vi "LinearBearingControl.vi"() -> ()   [LabVIEW 2012]
uses:
  stressTestTypeDef.ctl
  <vilib>/Utility/error.llb/DialogType.ctl
  allStatesTypeDef.ctl
  <vilib>/Utility/file.llb/Write To Spreadsheet File (DBL).vi
panel:
  out "sqrt(x)":dbl[](array[numeric])
  out "transposed array":dbl[][](array[numeric])
  in  "pulse/rev":u16(ring)=25600 items=["400"=400, "800"=800, "1600"=1600, "3200"=3200, "6400"=6400, "12800"=12800, "25600"=25600]
  out "concatenated string":string
  out "rigid body LED":bool
  out "strain rate":dbl
  in  "chain L0":i32=230
  out "mm/s (timed)":dbl
  in  "Direction":bool
  in  "Only Move Lin":bool
  out "writing data":bool
  out "stop sys":bool
  out "udp error out":errorcluster
  out "Voltages":dbl[][](array[numeric])
  in  "Start System":bool
  in  "Auto Bias":bool=TRUE
  in  "Unbias":bool
  in  "Bias":bool
  in  "Collect Data":bool=TRUE
  out "Measurement":dbl[][](graph) caption="F/T Data"
  out "Bias Vector":dbl[](array[numeric])
  in  "Timing parameters":T1={"Sample Rate"=1000.0, "Samples to Read"=100}
  in  "Transform":T2
  in  "Channel Parameters":T3={"First Channel"=1, "Number of Channels"=6, "DAQ Card"="Dev2", "Maximum Value"=10.0, "Minimum Value"=-10.0}
  in  "Sensor Parameters":T4={"Calibration File"=path "D:/ArduinoSmarticle/entangledSmarticle/FT21164.cal", "Force Units"="N", "Torque Units"="N-mm"}
  out "filenameOut":string
  in  "Optitrack Parameters":T5={"Optitrack IP"="130.207.141.229", "Optitrack Port"=1520, "timeout (sec)"=80}
  out "Data Output File":path
  in  "Output Folder":path=path "C:/Users/Administrator/Dropbox/expData/chainData"
  in  "Program Parameters":T7={"v"=2200, "Iters"=2, "Speed"=5, "Delay"=0.5, "H"=11.5, "SD"=10, "Name"="Stretch", "Type"=enum."FRACT ON"} {"Speed" min=0 max=49 step=5}
  out "strain %":dbl
  out "FT error out":errorcluster
  # "for 6 smarts\nSDmax ~ 170mm"
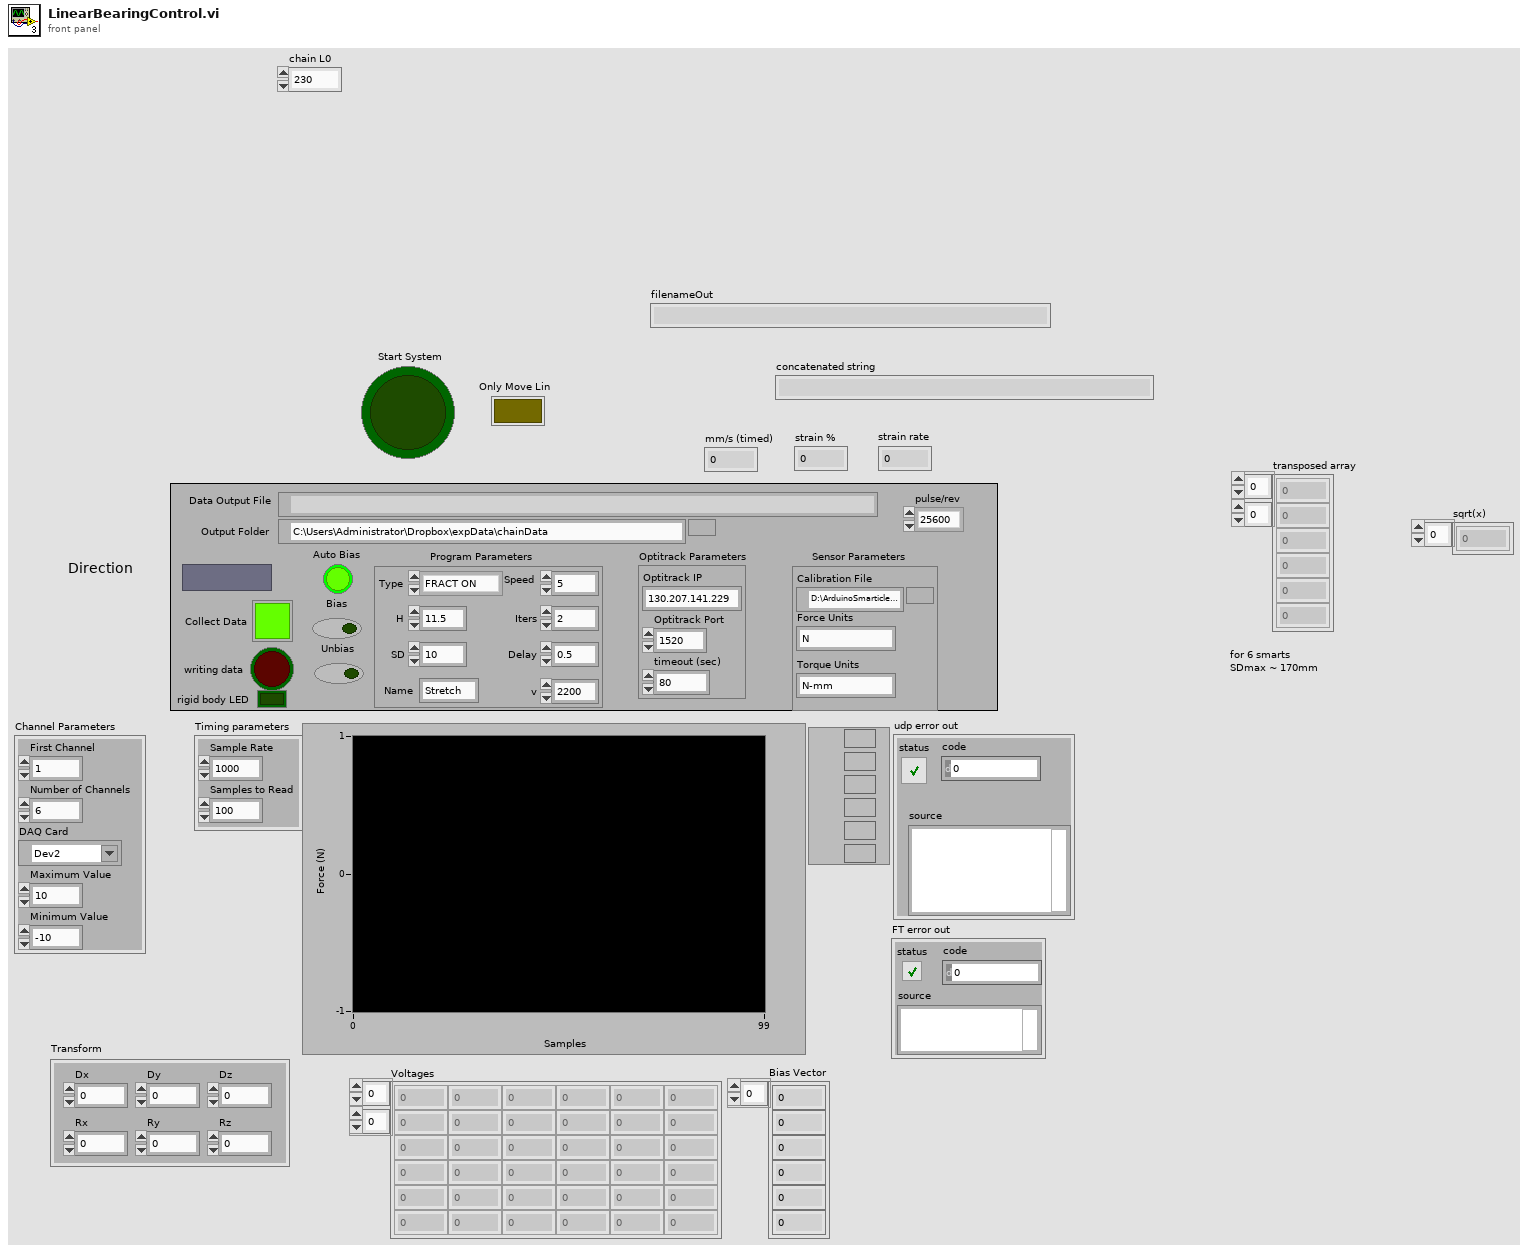
[diagram p1: front panel]
types:
  T1 = cluster{"Sample Rate":dbl, "Samples to Read":i32}
  T2 = cluster{"Dx":dbl, "Dy":dbl, "Dz":dbl, "Rx":dbl, "Ry":dbl, "Rz":dbl}
  T3 = cluster{"First Channel":i16, "Number of Channels":i16, "DAQ Card":tag, "Maximum Value":dbl, "Minimum Value":dbl}
  T4 = cluster{"Calibration File":path, "Force Units":string, "Torque Units":string}
  T5 = cluster{"Optitrack IP":string, "Optitrack Port":u16, "timeout (sec)":i32}
  T6 = typedef "stressTestTypeDef.ctl" = enum16{"OFF", "ON", "EXTEND", "SPRING", "FRACT ON", "SAC", "FRACT SAC"}
  T7 = cluster{"v":i32, "Iters":i32, "Speed":i32, "Delay":dbl, "H":dbl, "SD":i32, "Name":string, "Type":T6}
  T8 = cluster{"distance mm":i32, "Direction":bool, "device name":tag, "speed (mm/s)":i32, "pulse/rev":u16}
  T9 = typedef "DialogType.ctl" = u16
  T10 = cluster{"SD":i32, "Delay":dbl, "Speed":i32, "Iters":i32, "Type":T6, "timeout":i32}
  T11 = typedef "allStatesTypeDef.ctl" = enum16{"open udp", "start record", "recording", "move linear actuator", "end record", "close udp", "end"}
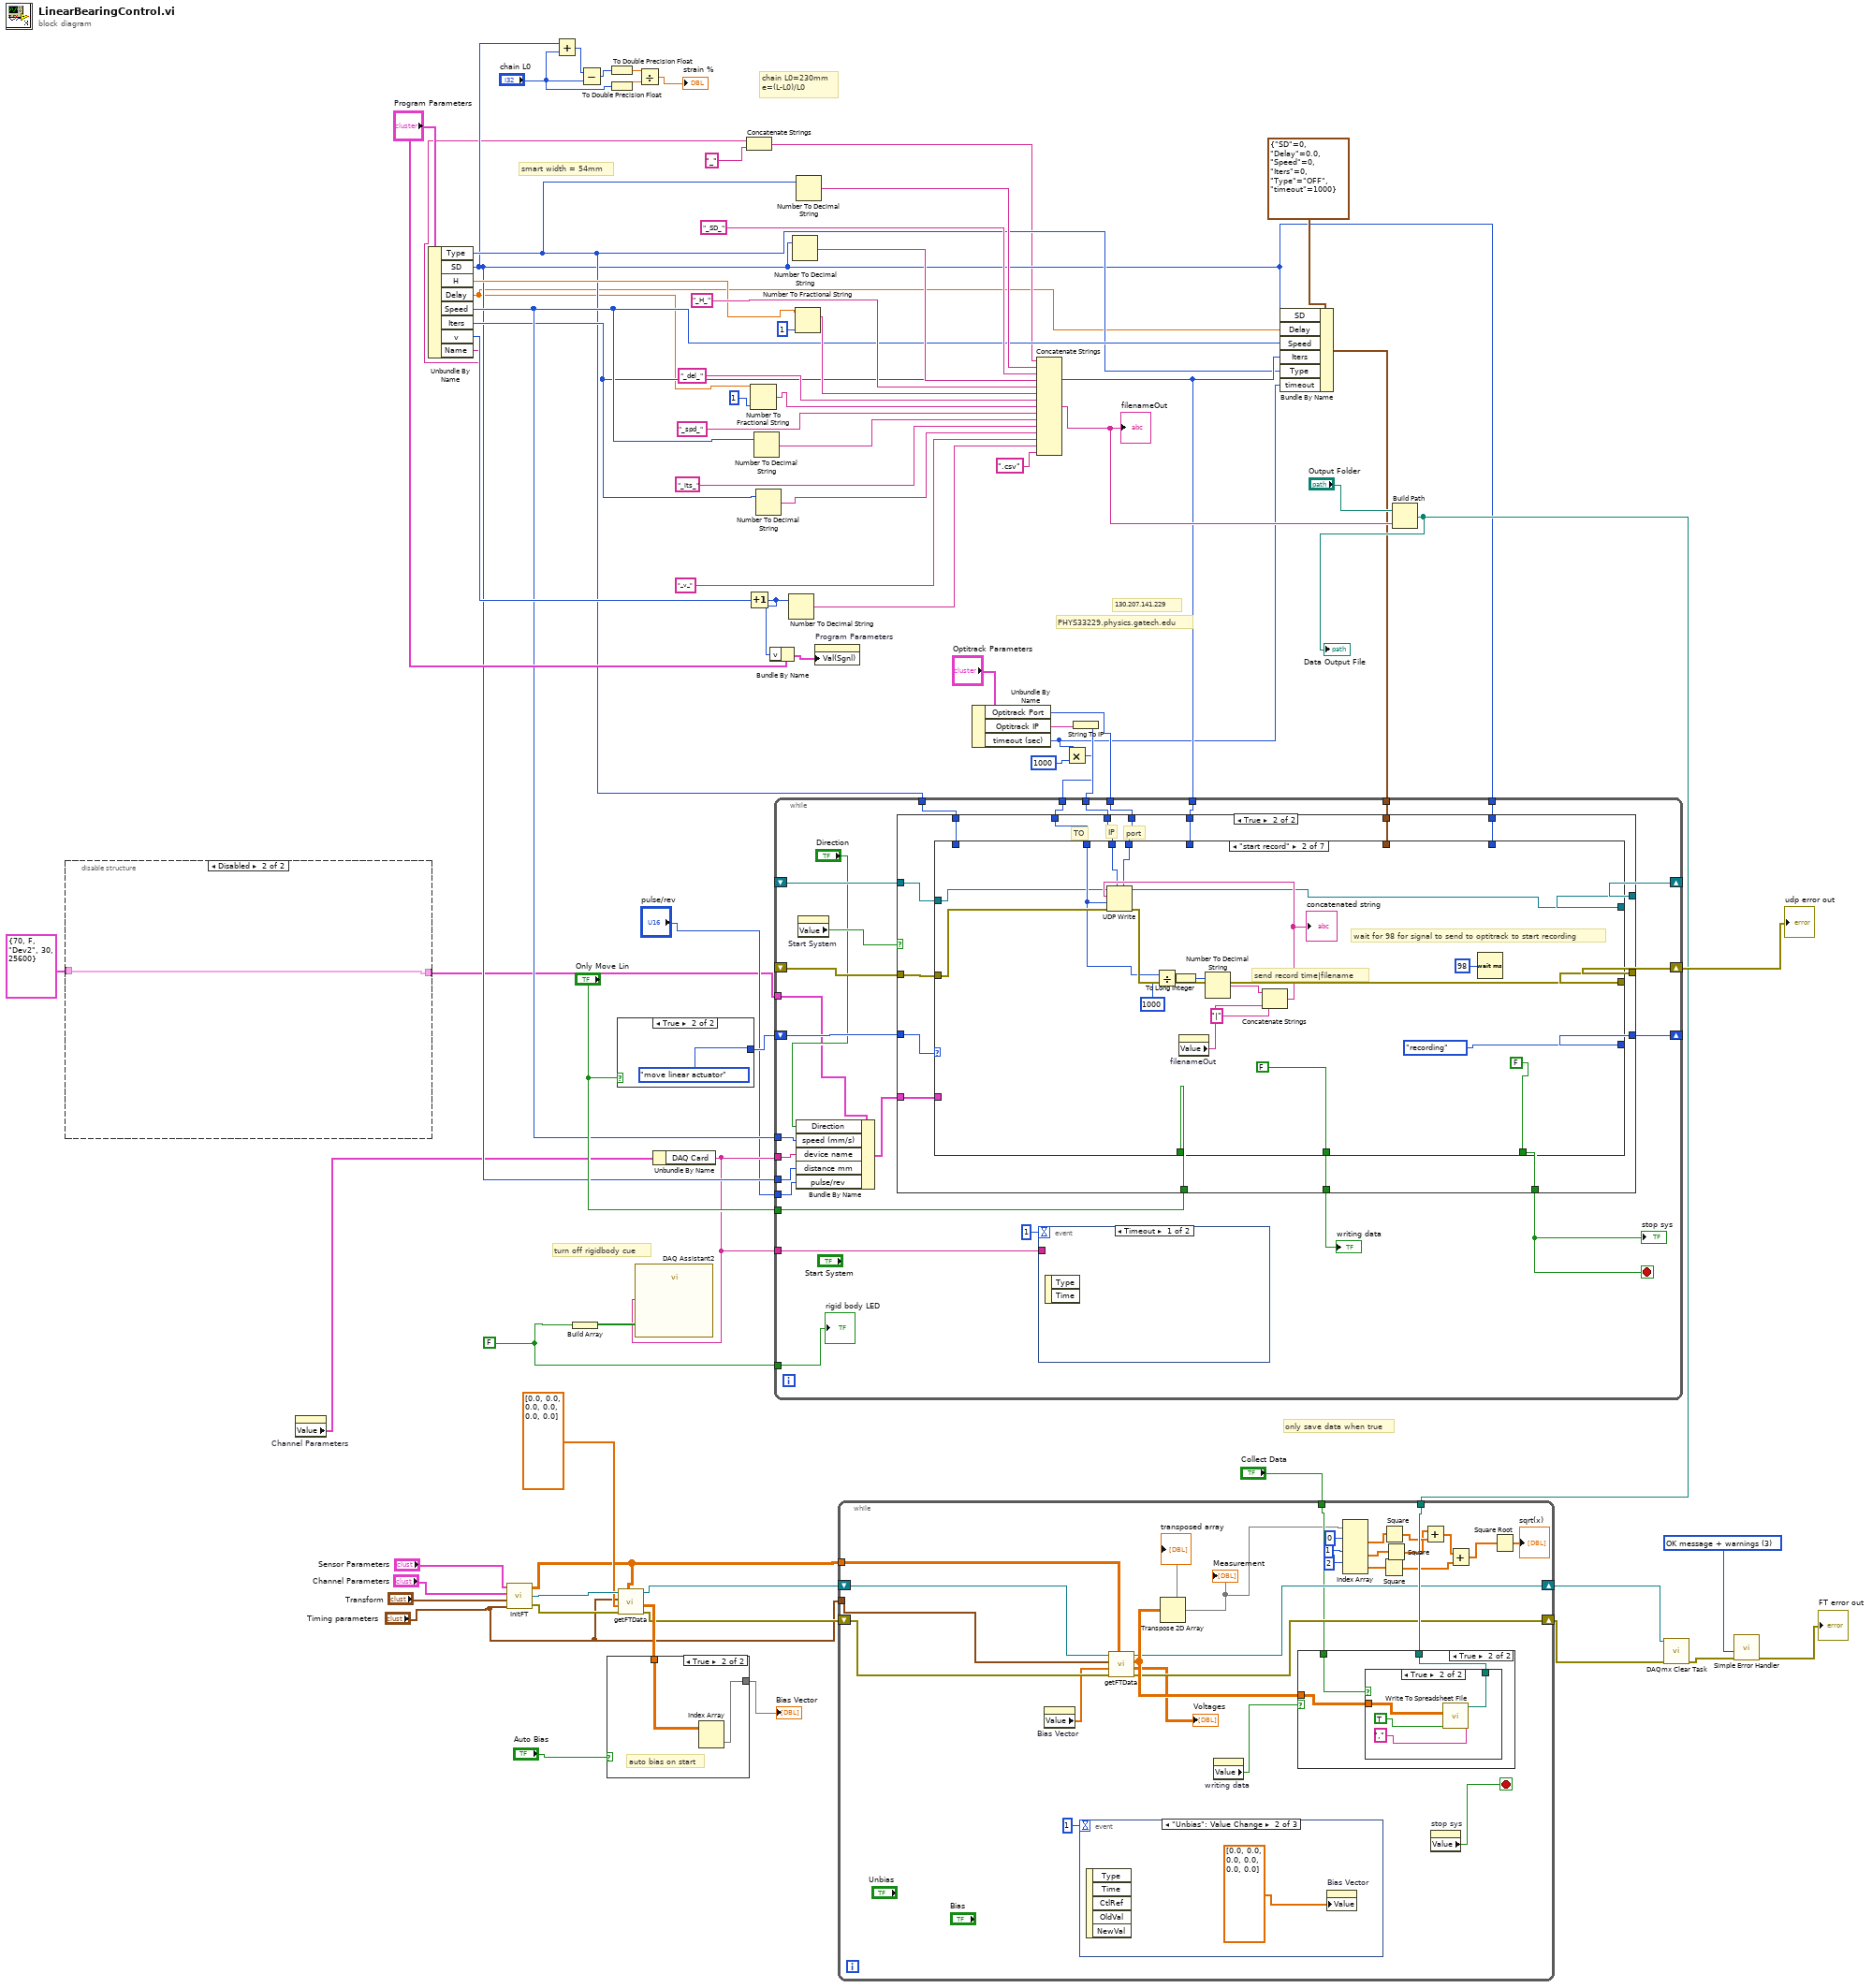
[diagram p0: block diagram]
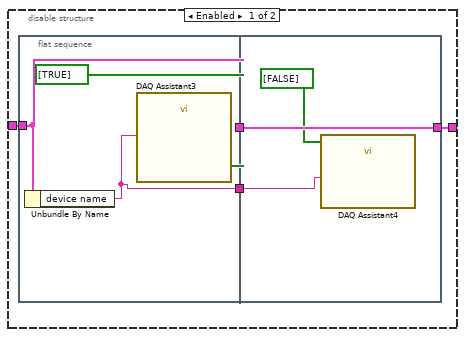
[diagram p2: hidden frame]
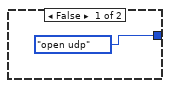
[diagram p3: hidden frame]
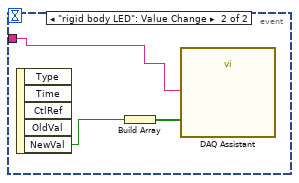
[diagram p4: hidden frame]
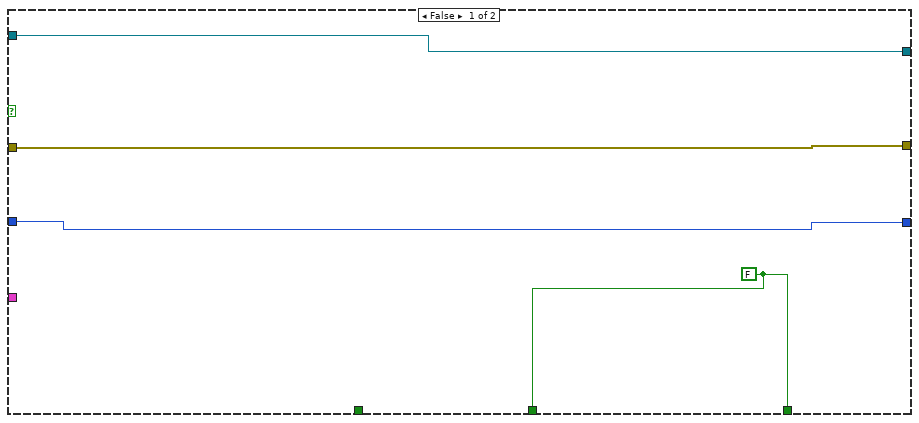
[diagram p5: hidden frame]
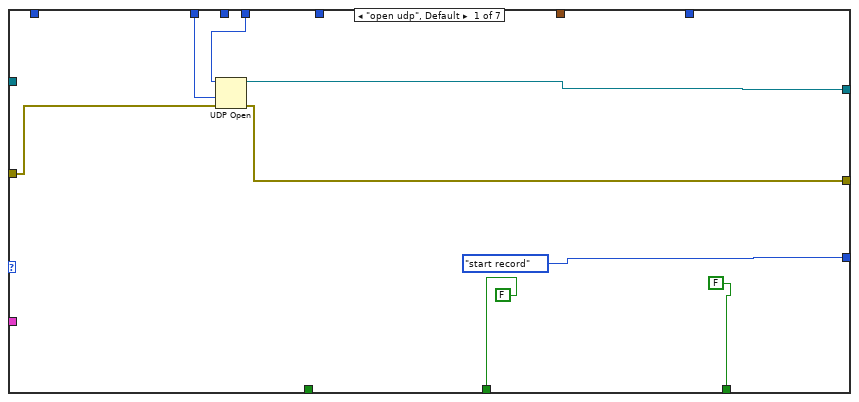
[diagram p6: hidden frame]
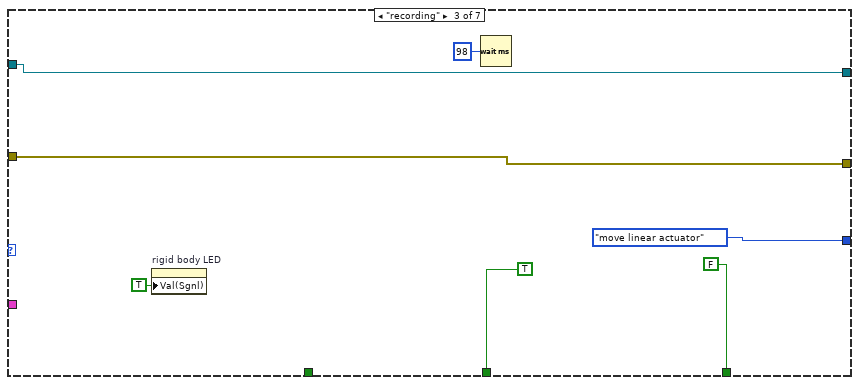
[diagram p7: hidden frame]
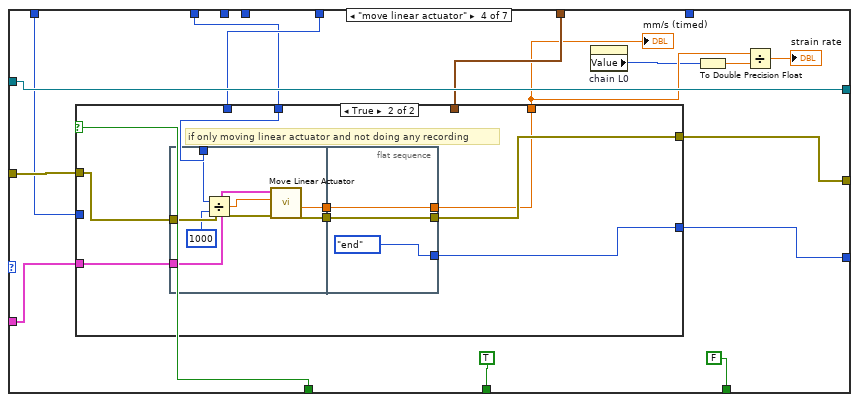
[diagram p8: hidden frame]
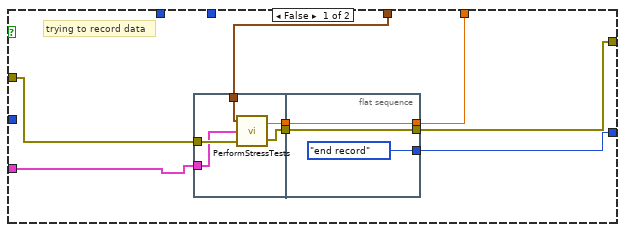
[diagram p9: hidden frame]
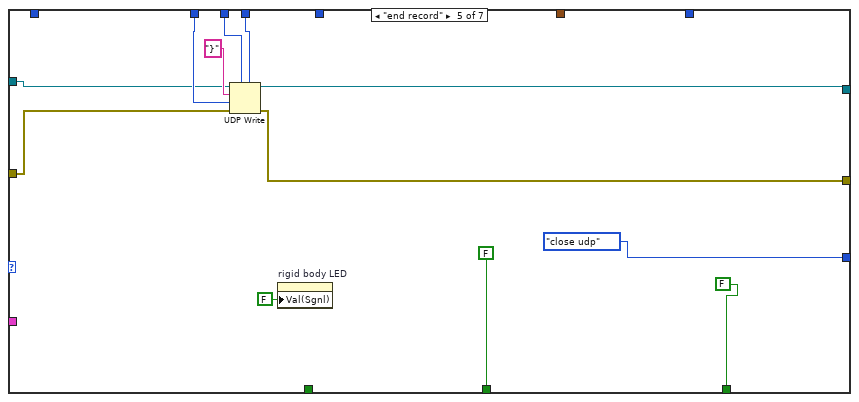
[diagram p10: hidden frame]
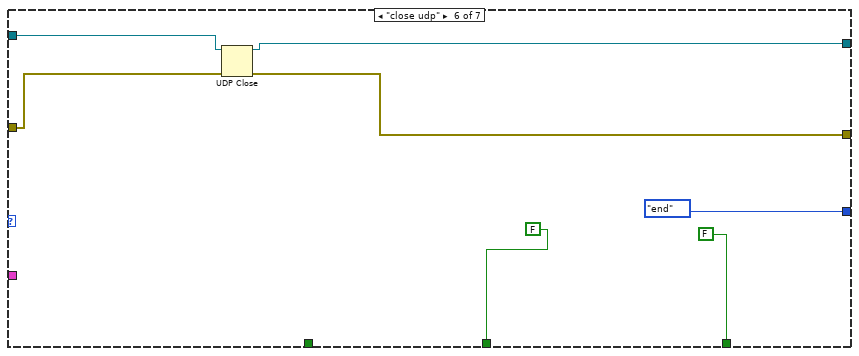
[diagram p11: hidden frame]
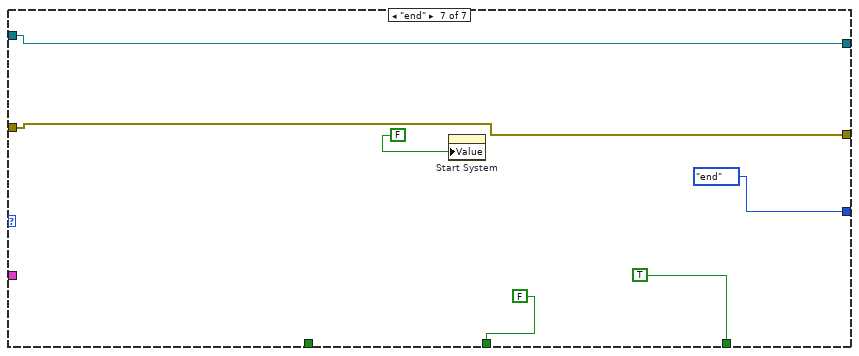
[diagram p12: hidden frame]
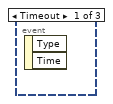
[diagram p13: hidden frame]
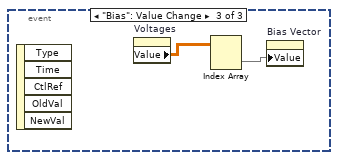
[diagram p14: hidden frame]
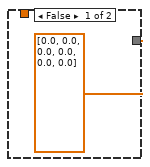
[diagram p17: hidden frame]
diagram:
  w13 = FALSE
  w46 = T9 3 items=["no dialog", "OK message", "continue or stop message", "OK message + warnings", "continue/stop + warnings"] ("type of dialog (OK msg:1)")
  # "turn off rigidbody cue"
  # "chain L0=230mm\ne=(L-L0)/L0"
  # "only save data when true"
  # "smart width = 54mm"
  # "PHYS33229.physics.gatech.edu"
  # "130.207.141.229"
  n1 = disable-structure shown="Disabled" {
    disable-tunnel: [w78 w87] -> w2
    disable-tunnel: T8 {"distance mm"=70, "Direction"=FALSE, "device name"="Dev2", "speed (mm/s)"=30, "pulse/rev"=25600} ("linear actuator info") -> [w77 w87]
    frame Enabled {
      n2 = flat-sequence {
        tunnel: w77 -> [w83]
        tunnel: [w83] -> w80
        tunnel: [w81] -> w79
        tunnel: [w86] -> w78
        tunnel: w80 -> [w86]
        tunnel: w79 -> [w85]
        frame #0 {
          n3 = Unbundle By Name(w83) -> ("device name"=w81:tag)
          n4 = call "DAQ Assistant3"("data"=bool[] [TRUE], "device name"=w81) -> ()  [unwired: 16 in, 2 out]
        }
        frame #1 {
          n5 = call "DAQ Assistant4"("data"=bool[] [FALSE], "device name"=w85) -> ()  [unwired: 16 in, 2 out]
        }
      }
    }
    frame Disabled {
    }
  }
  n6 = property on="Channel Parameters" class="Clust (strict)"() -> ("Value"=w12:T3)  [unwired: 2 in, 2 out]
  n7 = Unbundle By Name("Program Parameters") -> ("Type"=w23:T6, "SD"=w15:i32, "H"=w58:dbl, "Delay"=w5:dbl, "Speed"=w25:i32, "Iters"=w24:i32, "v"=w59:i32, "Name"=w8:string)
  n8 = call "InitFT.vi"("Timing parameters"="Timing parameters", "Transform"="Transform", "Channel Parameters"="Channel Parameters", "Sensor Parameters"="Sensor Parameters") -> ("error out"=w42:errorcluster, "task out"=w43:refnum<k21>, "Calibration Matrix"=w37:dbl[][])
  n9 = Add(x=w15, y="chain L0") -> (x+y=w21:i32)
  n10 = Build Array(w13) -> (w14:bool[])
  n11 = Subtract(x=w21, y="chain L0") -> (x-y=w20:i32)
  n12 = To Double Precision Float(number=w20) -> (double precision float=w18:dbl)
  n13 = To Double Precision Float(number="chain L0") -> (double precision float=w17:dbl)
  n14 = case shown="True" "Only Move Lin" {
    tunnel: [allStatesTypeDef."open udp" allStatesTypeDef."move linear actuator"] -> w76
    frame False {
    }
    frame True {
    }
  }
  n15 = call "getFTData.vi"("Transformed Calibration Matrix"=w37, "error in"=w42, "Bias Vector"=dbl[] [0.0, 0.0, 0.0, 0.0, 0.0, 0.0], "Timing parameters"="Timing parameters", "task in"=w43) -> ("error out"=w35:errorcluster, "Voltages"=w40:dbl[][], "task out 2"=w36:refnum<k21>)  [unwired: 1 out]
  n16 = case shown="True" "Auto Bias" {
    tunnel: w40 -> [_ w92]
    tunnel: [dbl[] [0.0, 0.0, 0.0, 0.0, 0.0, 0.0] w91] -> w33
    frame False {
    }
    frame True {
      # "auto bias on start"
      n17 = Index Array(array=w92) -> (element=w91:dbl[])  [unwired: 2 in]
    }
  }
  "Bias Vector" <- w33
  n18 = Divide(x=w18, y=w17) -> (x/y=→"strain %":dbl)
  n19 = Unbundle By Name(w12) -> ("DAQ Card"=w11:tag)
  n20 = call "DAQ Assistant2"("data"=w14, "device name"=w11) -> ()  [unwired: 16 in, 2 out]
  n21 = Concatenate Strings(w8, "_") -> (w9:string)
  n22 = Increment(x=w59) -> (x+1=w60:i32)
  n23 = Number To Fractional String(number=w5, precision (6)=i16 1) -> (F-format string=w3:string)  [unwired: 2 in]
  n24 = Number To Decimal String(number=w25) -> (decimal integer string=w64:string)  [unwired: 1 in]
  n25 = Number To Decimal String(number=w24) -> (decimal integer string=w62:string)  [unwired: 1 in]
  n26 = Bundle By Name(cluster="Program Parameters", "v"=w60) -> (w56:T7)
  n27 = Number To Decimal String(number=w60) -> (decimal integer string=w66:string)  [unwired: 1 in]
  n28 = Number To Decimal String(number=w15) -> (decimal integer string=w72:string)  [unwired: 1 in]
  n29 = Number To Fractional String(number=w58, precision (6)=i16 1) -> (F-format string=w69:string)  [unwired: 2 in]
  n30 = Number To Decimal String(number=w23) -> (decimal integer string=w74:string)  [unwired: 1 in]
  n31 = property on="Program Parameters" class="Clust (strict)"("Val(Sgnl)"=w56) -> ()  [unwired: 2 in, 2 out]
  n32 = Unbundle By Name("Optitrack Parameters") -> ("Optitrack Port"=w54:u16, "Optitrack IP"=w53:string, "timeout (sec)"=w7:i32)
  n33 = Concatenate Strings(w9, w74, "_SD_", w72, "_H_", w69, "_del_", w3, "_spd_", w64, "_its_", w62, "_v_", w66, ".csv") -> (w27:string)
  "filenameOut" <- w27
  n34 = Multiply(x=w7, y=1000) -> (x*y=w50:i32)
  n35 = String To IP(1:w53) -> (0:w52:u32)
  n36 = Bundle By Name(cluster=T10 {"SD"=0, "Delay"=0.0, "Speed"=0, "Iters"=0, "Type"=enum."OFF", "timeout"=1000}, "SD"=w15, "Delay"=w5, "Speed"=w25, "Iters"=w24, "Type"=w23, "timeout"=w7) -> (w22:T10)
  n37 = while {
    shift-right: [w119] -> w30
    shift-left: _ -> [w118]
    shift-right: [w116] -> _
    shift-left: w76 -> [w117]
    tunnel: w54 -> [w114]
    tunnel: w52 -> [w115]
    tunnel: w50 -> [w95]
    shift-right: [w113] -> _
    shift-left: _ -> [w112]
    tunnel: "Only Move Lin" -> [w109]
    tunnel: w25 -> [w106]
    tunnel: w15 -> [w97]
    tunnel: w23 -> [w105]
    tunnel: w24 -> [w104]
    tunnel: w22 -> [w103]
    tunnel: w15 -> [w101]
    tunnel: w13 -> [w100]
    tunnel: w11 -> [w98]
    tunnel: w11 -> [w96]
    tunnel: "pulse/rev" -> [w94]
    tunnel: w2 -> [w93]
    stop <- w111 stop-if-true
    n38 = Bundle By Name(cluster=w93, "Direction"="Direction", "speed (mm/s)"=w106, "device name"=w98, "distance mm"=w97, "pulse/rev"=w94) -> (w108:T8)
    n39 = property on="Start System" class="Bool (strict)"() -> ("Value"=w110:bool)  [unwired: 2 in, 2 out]
    n40 = case shown="True" w110 {
      tunnel: [w123 w143] -> w119
      tunnel: w118 -> [w123 w142]
      tunnel: w117 -> [w126 w141]
      tunnel: [w126 w140] -> w116
      tunnel: w115 -> [_ w139]
      tunnel: w114 -> [_ w132]
      tunnel: w95 -> [_ w138]
      tunnel: [w124 w137] -> w113
      tunnel: w112 -> [w124 w136]
      tunnel: [w125 w135] -> w102
      tunnel: [w125 w134] -> w111
      tunnel: w109 -> [_ w133]
      tunnel: w108 -> [_ w131]
      tunnel: w105 -> [_ w130]
      tunnel: w104 -> [_ w129]
      tunnel: w103 -> [_ w128]
      tunnel: w101 -> [_ w127]
      frame False {
        w125 = FALSE
      }
      frame True {
        # "IP"
        # "TO"
        # "port"
        n41 = case shown="\"start record\"" w141 {
          tunnel: w138 -> [w148 w161 _ w177 w234 _ _]
          tunnel: w142 -> [w149 w167 w172 w188 w238 w244 w246]
          tunnel: [w150 w168 w172 w187 w237 w245 w246] -> w143
          tunnel: [allStatesTypeDef."start record" allStatesTypeDef."recording" allStatesTypeDef."move linear actuator" w190 allStatesTypeDef."close udp" allStatesTypeDef."end" allStatesTypeDef."end"] -> w140
          tunnel: [FALSE FALSE FALSE FALSE FALSE FALSE TRUE] -> w134
          tunnel: w139 -> [_ w154 _ _ w228 _ _]
          tunnel: [w147 w157 w173 w189 w232 w243 w251] -> w137
          tunnel: w136 -> [_ w158 w173 w189 w231 w239 w251]
          tunnel: [FALSE FALSE TRUE TRUE FALSE FALSE FALSE] -> w135
          tunnel: w133 -> [_ _ _ w186 _ _ _]
          tunnel: w132 -> [w144 w153 _ _ w229 _ _]
          tunnel: w131 -> [_ _ _ w185 _ _ _]
          tunnel: w130 -> [_ _ _ w183 _ _ _]
          tunnel: w129 -> [_ _ _ w184 _ _ _]
          tunnel: w128 -> [_ _ _ w182 _ _ _]
          tunnel: w127 -> [_ _ _ _ _ _ _]
          frame "open udp", Default {
            n42 = UDP Open(8:w149, 9:w148, 11:w144) -> (port=w147:refnum<k16>, 0:w150:errorcluster)  [unwired: 2 in, 1 out]
          }
          frame "start record" {
            # "wait for 98 for signal to send to optitrack to start recording"
            # "send record time|filename"
            n43 = Divide(x=w161, y=1000) -> (x/y=w160:dbl)
            n44 = To Long Integer(number=w160) -> (32bit integer=w159:i32)
            n45 = property on="filenameOut" class="Str"() -> ("Value"=w165:string)  [unwired: 2 in, 2 out]
            n46 = Number To Decimal String(number=w159) -> (decimal integer string=w163:string)  [unwired: 1 in]
            n47 = Concatenate Strings(w163, "|" ("string"), w165) -> (w164:string)
            "concatenated string" <- w164
            n48 = UDP Write(address=w154, port or service name=w153, connection ID=w158, data in=w164, 8:w167, 9:w161) -> (error out=w168:errorcluster, 3:w157:refnum<k16>)
            n49 = Wait (ms)(milliseconds to wait=u32 98) -> ()  [unwired: 1 out]
          }
          frame "recording" {
            n50 = property on="rigid body LED" class="Bool (strict)"("Val(Sgnl)"=TRUE ("Value (Signaling)")) -> ()  [unwired: 2 in, 2 out]
            n51 = Wait (ms)(milliseconds to wait=u32 98) -> ()  [unwired: 1 out]
          }
          frame "move linear actuator" {
            n52 = case shown="True" w186 {
              tunnel: [w193 w210] -> w190
              tunnel: w188 -> [w197 w214]
              tunnel: [w196 w215] -> w187
              tunnel: w185 -> [w198 w216]
              tunnel: [w199 w213] -> w181
              tunnel: w184 -> [_ _]
              tunnel: w183 -> [_ _]
              tunnel: w182 -> [w200 _]
              tunnel: w177 -> [_ w209]
              frame False {
                # "trying to record data"
                n53 = flat-sequence {
                  tunnel: w200 -> [w205]
                  tunnel: w198 -> [w201]
                  tunnel: w197 -> [w203]
                  tunnel: [w204] -> w195
                  tunnel: [w202] -> w194
                  tunnel: w195 -> [w208]
                  tunnel: w194 -> [w207]
                  tunnel: [w208] -> w199
                  tunnel: [w207] -> w196
                  tunnel: [allStatesTypeDef."end record"] -> w193
                  frame #0 {
                    n54 = call "PerformStressTests.vi"("error in"=w203, "linear actuator info"=w201, "Test Info"=w205) -> ("error out"=w202:errorcluster, "mm/s (timed)"=w204:dbl)
                  }
                  frame #1 {
                  }
                }
              }
              frame True {
                # "if only moving linear actuator and not doing any recording"
                n55 = flat-sequence {
                  tunnel: w216 -> [w223]
                  tunnel: w214 -> [w221]
                  tunnel: [w222] -> w212
                  tunnel: [w220] -> w211
                  tunnel: w209 -> [w218]
                  tunnel: w212 -> [w226]
                  tunnel: w211 -> [w225]
                  tunnel: [w226] -> w215
                  tunnel: [w225] -> w213
                  tunnel: [allStatesTypeDef."end"] -> w210
                  frame #0 {
                    n56 = Divide(x=w218, y=1000) -> (x/y=w217:dbl)
                    n57 = call "Move Linear Actuator.vi"("error in"=w221, "timeout"=w217, "linear actuator info"=w223) -> ("error out"=w222:errorcluster, "mm/s (timed)"=w220:dbl)  [unwired: 1 in, 1 out]
                  }
                  frame #1 {
                  }
                }
              }
            }
            "mm/s (timed)" <- w181
            n58 = property on="chain L0" class="DigNum (strict)"() -> ("Value"=w180:i32)  [unwired: 2 in, 2 out]
            n59 = To Double Precision Float(number=w180) -> (double precision float=w179:dbl)
            n60 = Divide(x=w181, y=w179) -> (x/y=→"strain rate":dbl)
          }
          frame "end record" {
            n61 = UDP Write(address=w228, port or service name=w229, connection ID=w231, data in="}", 8:w238, 9:w234) -> (error out=w237:errorcluster, 3:w232:refnum<k16>)
            n62 = property on="rigid body LED" class="Bool (strict)"("Val(Sgnl)"=FALSE ("Value (Signaling)")) -> ()  [unwired: 2 in, 2 out]
          }
          frame "close udp" {
            n63 = UDP Close(connection ID=w239, 8:w244) -> (connection ID out=w243:refnum<k16>, error out=w245:errorcluster)
          }
          frame "end" {
            n64 = property on="Start System" class="Bool (strict)"("Value"=FALSE) -> ()  [unwired: 2 in, 2 out]
          }
        }
      }
    }
    "stop sys" <- w111
    "writing data" <- w102
    n65 = event shown="[0] Timeout" {
      selector: _ -> [_ _]
      dyn-events: _ -> [_ _]
      timeout: 1 -> [_ _]
      tunnel: w96 -> [_ w120]
      event Timeout {
        n66 = event-data() -> ()  [unwired: 1 in, 2 out]
      }
      event "rigid body LED": Value Change {
        n67 = event-data() -> ("NewVal"=w121:bool)  [unwired: 1 in, 4 out]
        n68 = Build Array(w121) -> (w122:bool[])
        n69 = call "DAQ Assistant"("data"=w122, "device name"=w120) -> ()  [unwired: 16 in, 2 out]
      }
    }
    "rigid body LED" <- w100
  }
  "udp error out" <- w30
  n70 = Build Path(base path="Output Folder", name or relative path=w27) -> (appended path=w29:path)
  "Data Output File" <- w29
  n71 = while {
    tunnel: w29 -> [w277]
    tunnel: "Collect Data" -> [w266]
    tunnel: w37 -> [w274]
    shift-right: [w276] -> w32
    shift-left: w36 -> [w273]
    shift-right: [w271] -> w31
    shift-left: w35 -> [w275]
    tunnel: "Timing parameters" -> [w272]
    stop <- w267 stop-if-true
    n72 = property on="Bias Vector" class="Arr (strict)"() -> ("Value"=w270:dbl[])  [unwired: 2 in, 2 out]
    n73 = event shown="[1] \"Unbias\": Value Change" {
      selector: _ -> [_ _ _]
      dyn-events: _ -> [_ _ _]
      timeout: 1 -> [_ _ _]
      event Timeout {
        n74 = event-data() -> ()  [unwired: 1 in, 2 out]
      }
      event "Unbias": Value Change {
        n75 = event-data() -> ()  [unwired: 1 in, 5 out]
        n76 = property on="Bias Vector" class="Arr (strict)"("Value"=dbl[] [0.0, 0.0, 0.0, 0.0, 0.0, 0.0]) -> ()  [unwired: 2 in, 2 out]
      }
      event "Bias": Value Change {
        n77 = event-data() -> ()  [unwired: 1 in, 5 out]
        n78 = property on="Voltages" class="Arr (strict)"() -> ("Value"=w280:dbl[][])  [unwired: 2 in, 2 out]
        n79 = Index Array(array=w280) -> (element=w281:dbl[])  [unwired: 2 in]
        n80 = property on="Bias Vector" class="Arr (strict)"("Value"=w281) -> ()  [unwired: 2 in, 2 out]
      }
    }
    n81 = call "getFTData.vi"("Transformed Calibration Matrix"=w274, "error in"=w275, "Bias Vector"=w270, "Timing parameters"=w272, "task in"=w273) -> ("error out"=w271:errorcluster, "Voltages"=→"Voltages":dbl[][], "F/T"=w278:dbl[][], "task out 2"=w276:refnum<k21>)
    n82 = Transpose 2D Array(2D array=w278) -> (transposed array=w259:dbl[][])
    "Measurement" <- w259
    "transposed array" <- w259
    n83 = property on="writing data" class="Bool (strict)"() -> ("Value"=w265:bool)  [unwired: 2 in, 2 out]
    n84 = case shown="True" w265 {
      tunnel: w278 -> [_ w284]
      tunnel: w277 -> [_ w283]
      tunnel: w266 -> [_ w282]
      frame False {
      }
      frame True {
        n85 = case shown="True" w282 {
          tunnel: w284 -> [_ w288]
          tunnel: w283 -> [_ w287]
          frame False {
          }
          frame True {
            n86 = call-poly <vilib>:"Write To Spreadsheet File.vi"("delimiter (\\t)"=",", "append to file? (new file:F)"=TRUE, "2D data"=w288, "file path (dialog if empty)"=w287) -> ()  [unwired: 4 in, 1 out]
          }
        }
      }
    }
    n87 = Index Array(array=w259, index (row) #1=0 ("index"), index (row) #2=1 ("index"), index (row) #3=2 ("index")) -> (element #1=w258:dbl[], element #2=w261:dbl[], element #3=w260:dbl[])  [unwired: 3 in]
    n88 = Square(x=w260) -> (x^2=w254:dbl[])
    n89 = Square(x=w258) -> (x^2=w257:dbl[])
    n90 = Square(x=w261) -> (x^2=w256:dbl[])
    n91 = Add(x=w256, y=w257) -> (x+y=w255:dbl[])
    n92 = property on="stop sys" class="Bool (strict)"() -> ("Value"=w267:bool)  [unwired: 2 in, 2 out]
    n93 = Add(x=w255, y=w254) -> (x+y=w253:dbl[])
    n94 = Square Root(x=w253) -> (sqrt(x)=→"sqrt(x)":dbl[])
  }
  n95 = call <vilib>:"DAQmx Clear Task.vi"("task in"=w32, "error in"=w31) -> ("error out"=w44:errorcluster)  [unwired: 13 in]
  n96 = call <vilib>:"Simple Error Handler.vi"("type of dialog (OK msg:1)"=w46, "error in (no error)"=w44) -> ("error out"=→"FT error out":errorcluster)  [unwired: 3 in, 4 out]
